vi "Configure Setpoint Window.vi"(8 "error in (no error)":errorcluster, 9 "Setpoint Window (2)":dbl=2.0 min=0.1 max=9.9 step=1.0, 11 "VISA resource name":refnum<visa-resource-name>) -> (0 "error out":errorcluster, 3 "VISA resource name out":refnum<visa-resource-name>)   [LabVIEW 2010, in "Temptronic TP04300.lvlib"]
doc: "This VI configures the setpoint window.\n\n<b>Setpoint temperature window</b>\nValid Range: 0.1 to 9.9 \nDefault Value: 2.0\n\nNote: The window is the maximum positive or negative deviation from \nthe temperature setpoint allowable for an \"at temperature\" condition."
uses:
  Temptronic TP04300.lvlib
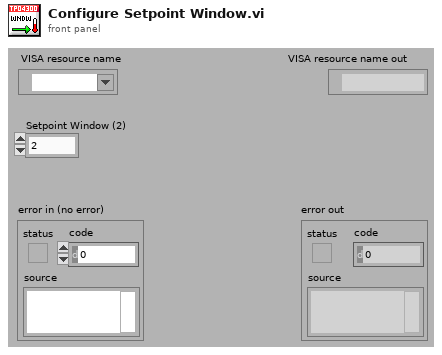
[diagram p1: front panel]
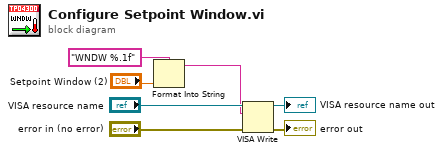
[diagram p0: block diagram]
diagram:
  n1 = Format Into String(format string="WNDW %.1f" ("multi-line string"), "Setpoint Window (2)") -> (resulting string=w3:string)  [unwired: 2 in, 1 out]
  n2 = VISA Write(VISA resource name="VISA resource name", write buffer=w3, error in (no error)="error in (no error)") -> (VISA resource name out=→"VISA resource name out":refnum<visa-resource-name>, error out=→"error out":errorcluster)  [unwired: 1 out]
